vi "AO Python Interface.vi"(7 "Calling VI Ref":refnum<vi>) -> ()   [LabVIEW 2016]
uses:
  AO Python Controls/LabView Python Notifier Element.ctl
  AO Python Controls/AO Python Actions.ctl
  AO Python Controls/AO Python Data Type.ctl
  AO Python Controls/AO Python Units.ctl
  AO Python Controls/AO Python Vector Type.ctl
  Hardware Configuration/Hardware Configuration Controls/Device Type.ctl
  Hardware Configuration/Hardware Configuration Controls/Device Function.ctl
  Device Library/AOTF and AOM/AOTF Controls/AOTF Actions.ctl
panel:
  in  "Quit":bool
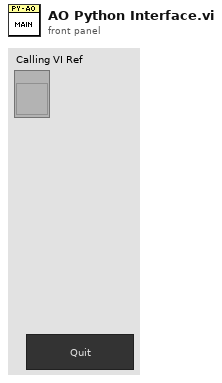
[diagram p1: front panel]
types:
  T1 = typedef "AO Python Actions.ctl" = enum16{"Error Check", "Query Commands", "Run Update", "Run Sensorless", "Wait for Command", "Get Image", "Update DM", "Get Status", "Quit"}
  T2 = typedef "LabView Python Notifier Element.ctl" = cluster{"Actions":T1, "Received?":bool, "Running?":bool, "AO Data":T3, "Command List":string[], "Python Status":string, "Error":errorcluster}
  T3 = typedef "AO Python Data Type.ctl" = cluster{"LV Command":string, "Vector":dbl[], "Flat On?":i32, "Units":T4, "Vector Type":T5}
  T4 = typedef "AO Python Units.ctl" = enum16{"rad", "nm"}
  T5 = typedef "AO Python Vector Type.ctl" = enum16{"Zernike", "Actuators", "Zernike High NA", "DM Modes"}
  T6 = typedef "Device Function.ctl" = enum16{"Primary", "Secondary", "Overview", "Wide Field Drift Correction", "642 nm Excitation", "560 nm Excitation", "546 nm Excitation", "488 nm Excitation", "405 nm Excitation", "Objective Drift Correction", "Objective XY", "Objective Z", "Sample XY", "Sample Coarse Z", "Sample Z", "4Pi Lower", "4Pi Upper", "Adj Cavity"}
  T7 = typedef "Device Type.ctl" = enum16{"AOTF", "Camera", "Deformable Mirror", "Laser", "Shutter", "Stage"}
  T8 = typedef "AOTF Actions.ctl" = enum16{"Error Check", "Blank", "Line On/Off", "Set Power", "Status", "Quit"}
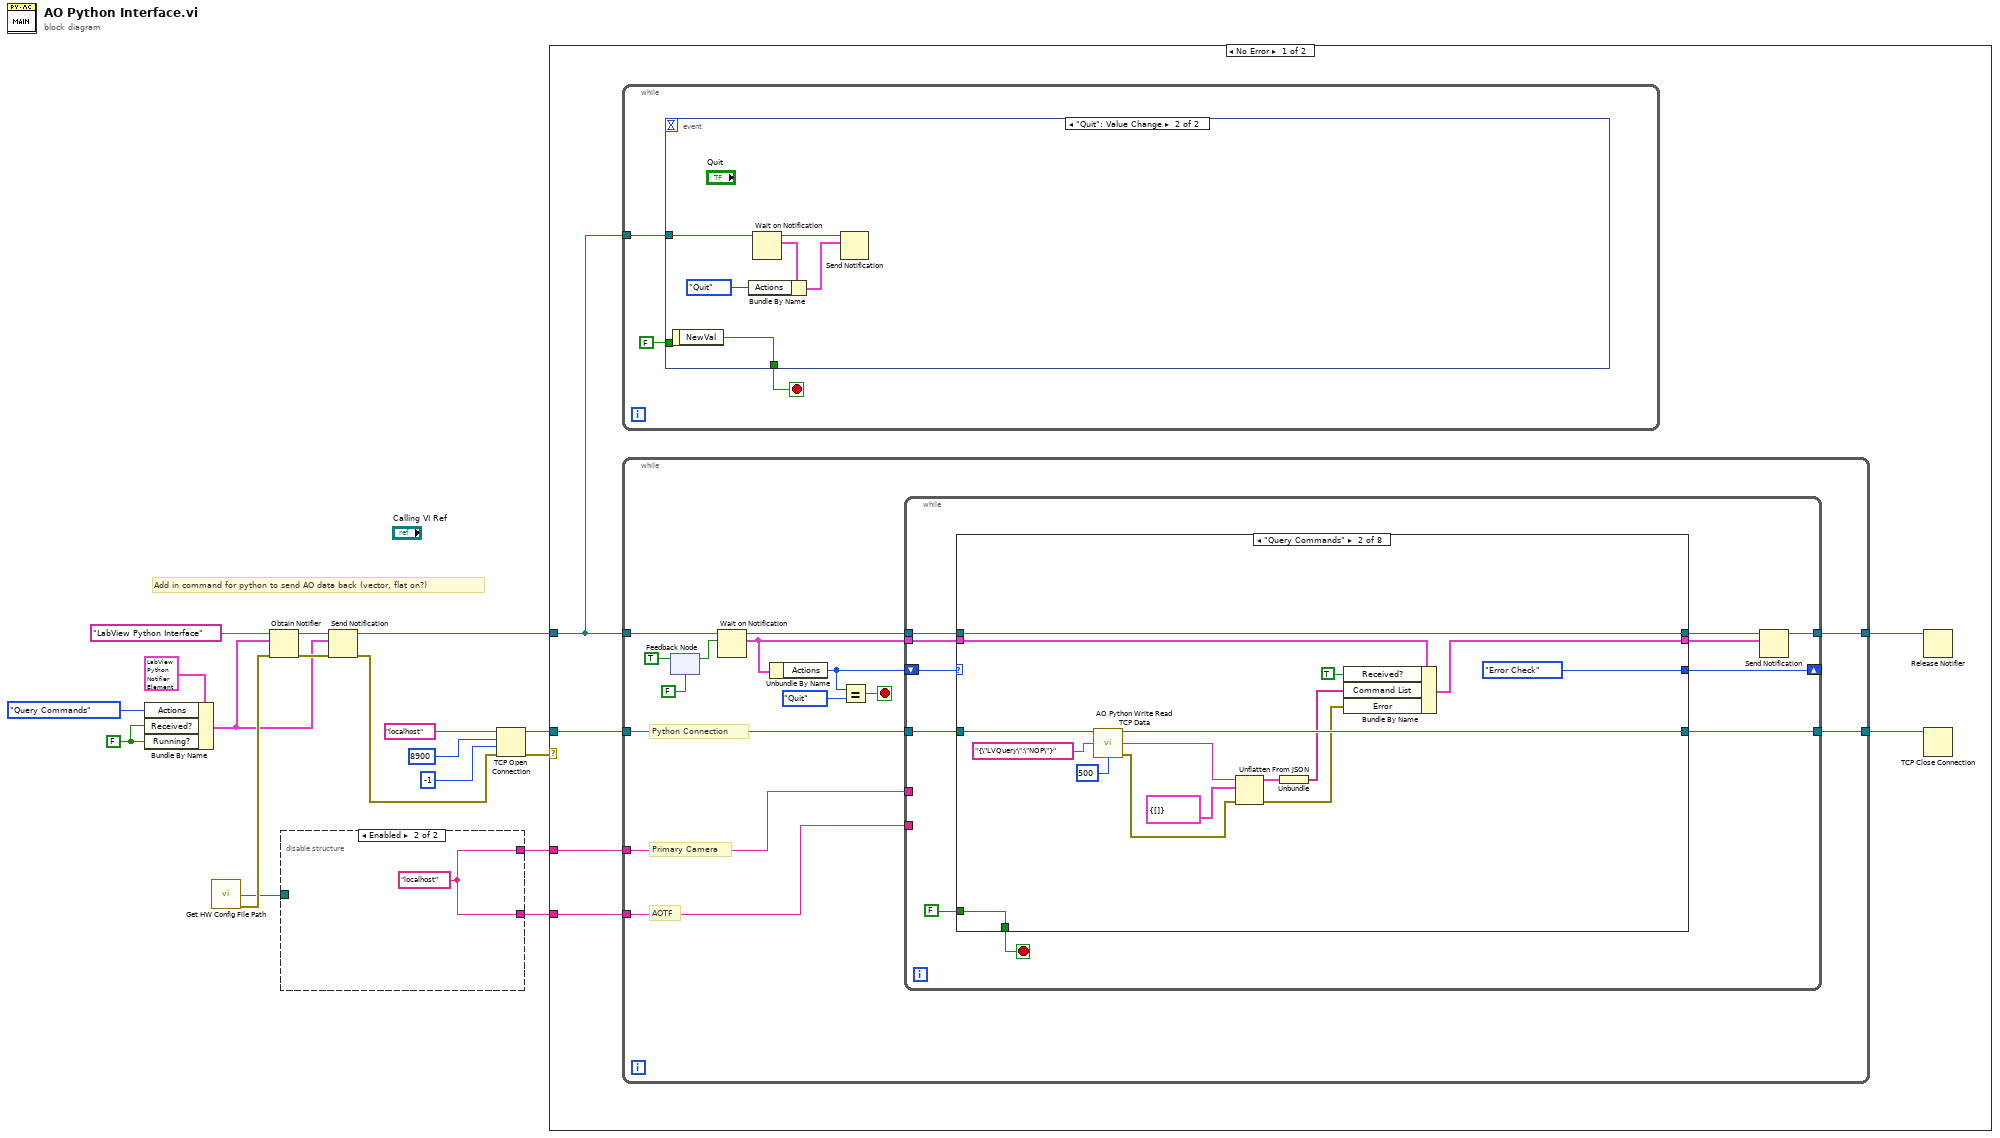
[diagram p0: block diagram]
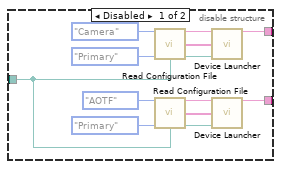
[diagram p2: hidden frame]
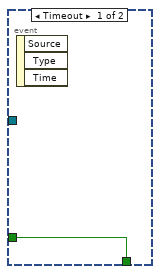
[diagram p3: hidden frame]
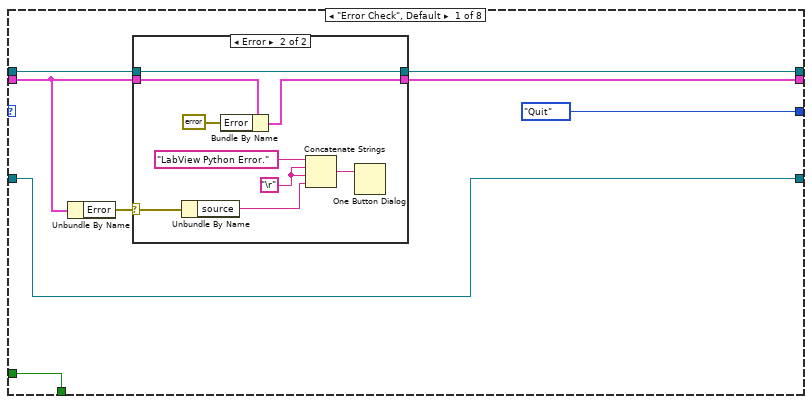
[diagram p4: hidden frame]
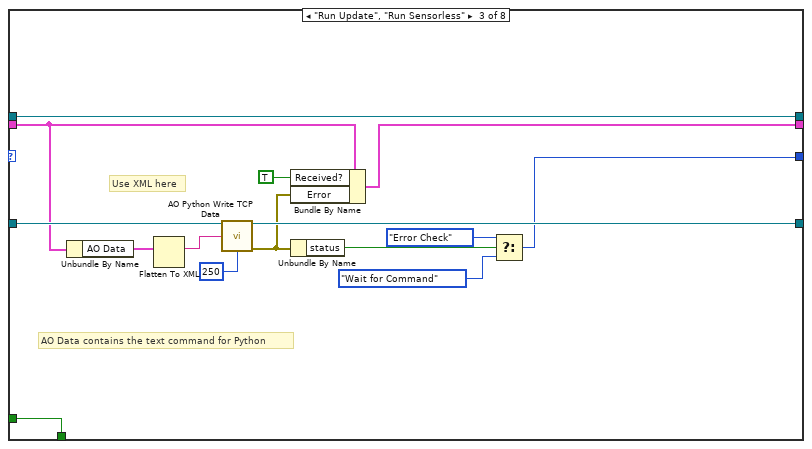
[diagram p6: hidden frame]
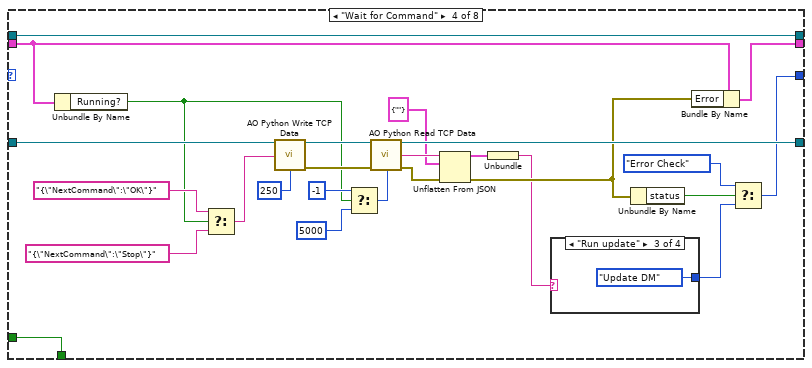
[diagram p7: hidden frame]
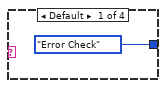
[diagram p8: hidden frame]
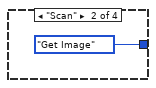
[diagram p9: hidden frame]
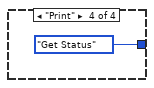
[diagram p10: hidden frame]
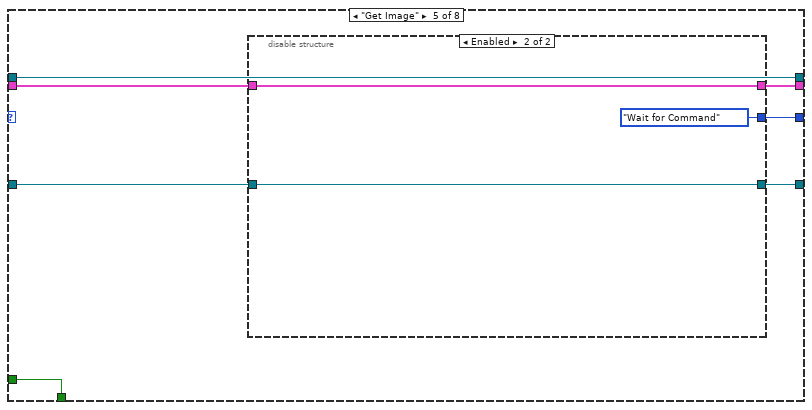
[diagram p11: hidden frame]
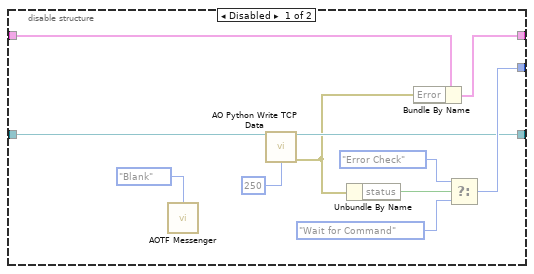
[diagram p12: hidden frame]
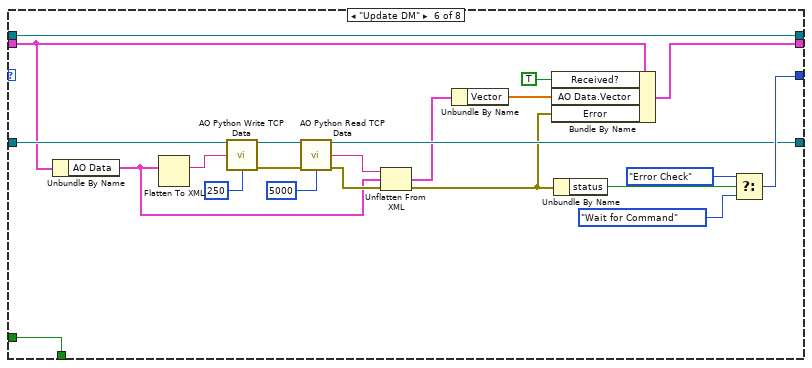
[diagram p13: hidden frame]
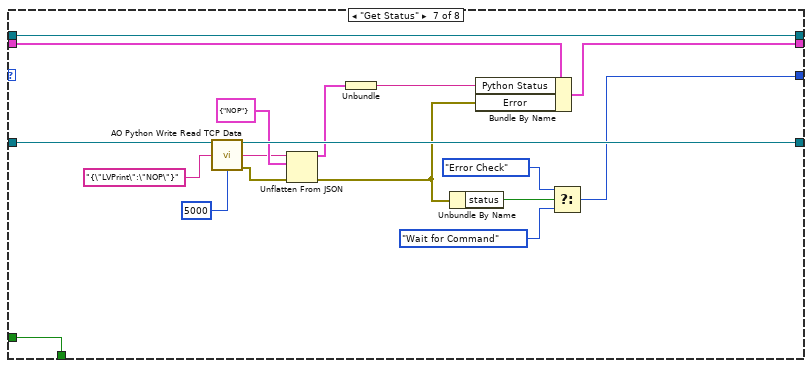
[diagram p14: hidden frame]
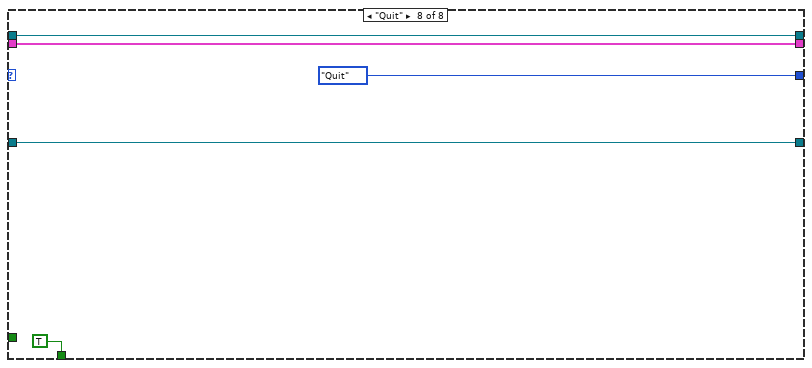
[diagram p15: hidden frame]
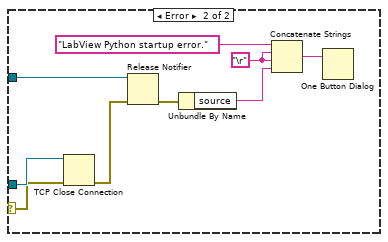
[diagram p16: hidden frame]
diagram:
  w3 = FALSE ("Received?")
  # "Add in command for python to send AO data back (vector, flat on?)"
  n1 = Bundle By Name(cluster=T2 {"Actions"=enum."Query Commands", "Received?"=FALSE, "Running?"=FALSE, "AO Data"={"LV Command"="", "Vector"=[], "Flat On?"=1, "Units"=enum."rad", "Vector Type"=enum."Zernike"}, "Command List"=[], "Python Status"="", "Error"={"status"=FALSE, "code"=0, "source"=""}} ("LabView Python Notifier Element"), "Actions"=AO_Python_Actions."Query Commands", "Received?"=w3, "Running?"=w3) -> (w1:T2)
  n2 = call "Get HW Config File Path.vi"() -> ("File Path"=w6:path, "Error"=w7:errorcluster)  [unwired: 14 in]
  n3 = Obtain Notifier(name (unnamed)="LabView Python Interface", notification data type=w1, error in (no error)=w7) -> (notifier out=w13:refnum<notifier>, error out=w11:errorcluster)  [unwired: 1 in, 1 out]
  n4 = disable-structure shown="Enabled" {
    disable-tunnel: [w26 w32] -> w8
    disable-tunnel: w6 -> [w20 _]
    disable-tunnel: [w19 w32] -> w5
    frame Disabled {
      n5 = call "Read Configuration File.vi"("Device Type"=Device_Type."Camera", "Device Function"=Device_Function."Primary", "Config File Path"=w20) -> ("Unique Notifier Name"=w31:string, "Device Ports/IDs/Channels"=w30:string[], "Device Engine Path"=w29:path)  [unwired: 9 in, 1 out]
      n6 = call "Read Configuration File.vi"("Device Type"=Device_Type."AOTF", "Device Function"=Device_Function."Primary", "Config File Path"=w20) -> ("Unique Notifier Name"=w21:string, "Device Ports/IDs/Channels"=w22:string[], "Device Engine Path"=w23:path)  [unwired: 9 in, 1 out]
      n7 = call "Device Launcher.vi"("Notifier Name"=w31, "Device Ports/IDs/Channels"=w30, "Device Engine Path"=w29) -> ("Notifier Name"=w26:string)  [unwired: 11 in, 1 out]
      n8 = call "Device Launcher.vi"("Notifier Name"=w21, "Device Ports/IDs/Channels"=w22, "Device Engine Path"=w23) -> ("Notifier Name"=w19:string)  [unwired: 11 in, 1 out]
    }
    frame Enabled {
      w32 = "localhost" ("address")
    }
  }
  n9 = Send Notification(notification=w1, notifier=w13, error in (no error)=w11) -> (notifier out=w12:refnum<notifier>, error out=w10:errorcluster)
  n10 = TCP Open Connection(address="localhost", remote port or service name=u16 8900, timeout ms (60000)=-1, error in (no error)=w10) -> (connection ID=w15:refnum<k5>, error out=w9:errorcluster)  [unwired: 1 in]
  n11 = case shown="No Error" w9 {
    selector: w9 -> [_ w226]
    tunnel: w15 -> [w38 w227]
    tunnel: w12 -> [w33 w228]
    tunnel: w8 -> [w37 _]
    tunnel: w5 -> [w34 _]
    frame No Error {
      n12 = while {
        tunnel: w33 -> [w39]
        stop <- w41 stop-if-true
        n13 = event shown="[1] \"Quit\": Value Change" {
          selector: _ -> [_ _]
          dyn-events: _ -> [_ _]
          timeout: _ -> [_ _]
          tunnel: [w42 w48] -> w41
          tunnel: FALSE -> [w42 _]
          tunnel: w39 -> [_ w47]
          event Timeout {
            n14 = event-data() -> ()  [unwired: 1 in, 3 out]
          }
          event "Quit": Value Change {
            n15 = event-data() -> ("NewVal"=w48:bool)  [unwired: 1 in]
            n16 = Wait on Notification(notifier=w47) -> (notifier out=w46:refnum<notifier>, notification=w45:T2)  [unwired: 3 in, 2 out]
            n17 = Bundle By Name(cluster=w45, "Actions"=AO_Python_Actions."Quit") -> (w43:T2)
            n18 = Send Notification(notification=w43, notifier=w46) -> ()  [unwired: 1 in, 2 out]
          }
        }
      }
      n19 = while {
        tunnel: w38 -> [w53]
        tunnel: w33 -> [w62]
        tunnel: w37 -> [w52]
        tunnel: [w51] -> w35
        tunnel: [w50] -> w36
        tunnel: w34 -> [w49]
        stop <- w58 stop-if-true
        # "AOTF"
        # "Primary Camera"
        # "Python Connection"
        n20 = feedback-in #1(TRUE) -> ()
        n21 = feedback #1(FALSE) -> (w55:bool)
        n22 = Wait on Notification(notifier=w62, ignore previous (F)=w55) -> (notifier out=w60:refnum<notifier>, notification=w54:T2)  [unwired: 2 in, 2 out]
        n23 = Unbundle By Name(w54) -> ("Actions"=w59:T1)
        n24 = Equal?(x=w59, y=AO_Python_Actions."Quit") -> (x = y?=w58:bool)
        n25 = while {
          tunnel: w60 -> [w71]
          shift-right: [w70] -> _
          shift-left: w59 -> [w73]
          tunnel: w54 -> [w72]
          tunnel: w53 -> [w68]
          tunnel: w52 -> [_]
          tunnel: [w66] -> w51
          tunnel: [w64] -> w50
          tunnel: w49 -> [_]
          stop <- w69 stop-if-true
          n26 = case shown="\"Query Commands\"" w73 {
            tunnel: w72 -> [w80 w98 w116 w133 w158 w182 w207 w215]
            tunnel: w71 -> [w81 w100 w120 w141 w159 w189 w213 w216]
            tunnel: [AO_Python_Actions."Quit" ("y") AO_Python_Actions."Error Check" ("y") w109 w134 w156 w188 w205 AO_Python_Actions."Quit" ("y")] -> w70
            tunnel: [w78 w108 w123 w149 w160 w175 w214 TRUE] -> w69
            tunnel: w68 -> [w76 w107 w122 w148 w155 w191 w212 w217]
            tunnel: FALSE -> [w78 w108 w123 w149 w160 w175 w214 _]
            tunnel: [w76 w106 w117 w136 w154 w185 w210 w217] -> w66
            tunnel: [w77 w100 w120 w141 w159 w189 w213 w216] -> w65
            tunnel: [w75 w97 w110 w132 w157 w190 w206 w215] -> w63
            frame "Error Check", Default {
              n27 = Unbundle By Name(w80) -> ("Error"=w79:errorcluster)
              n28 = case shown="Error" w79 {
                selector: w79 -> [_ w87]
                tunnel: w80 -> [w82 w91]
                tunnel: [w83 w89] -> w77
                tunnel: w81 -> [w83 w89]
                tunnel: [w82 w88] -> w75
                frame No Error {
                }
                frame Error {
                  w85 = "\r"
                  n29 = Unbundle By Name(w87) -> ("source"=w84:string)
                  n30 = Bundle By Name(cluster=w91, "Error"=errorcluster {"status"=FALSE, "code"=0, "source"=""}) -> (w88:T2)
                  n31 = Concatenate Strings("LabView Python Error." ("string"), w85, w85, w84) -> (w92:string)
                  n32 = One Button Dialog(message=w92) -> ()  [unwired: 1 in, 1 out]
                }
              }
            }
            frame "Query Commands" {
              n33 = call "AO Python Write Read TCP Data.vi"("Connection ID"=w107, "Write String"="{\"LVQuery\":\"NOP\"}", "Timeout (ms)"=500) -> ("Connection ID (Dup)"=w106:refnum<k5>, "Read String"=w101:string, "Error Out"=w99:errorcluster)  [unwired: 10 in]
              n34 = Unflatten From JSON(JSON string=w101, type and defaults=cluster{string[]} {[]}, error in (no error)=w99) -> (value=w103:cluster{string[]}, error out=w95:errorcluster)  [unwired: 4 in]
              n35 = Unbundle(w103) -> (w96:string[])
              n36 = Bundle By Name(cluster=w98, "Received?"=TRUE, "Command List"=w96, "Error"=w95) -> (w97:T2)
            }
            frame "Run Update", "Run Sensorless" {
              # "Use XML here"
              # "AO Data contains the text command for Python"
              n37 = Unbundle By Name(w116) -> ("AO Data"=w119:T3)
              n38 = Flatten To XML(anything=w119) -> (xml string=w118:string)
              n39 = call "AO Python Write TCP Data.vi"("Connection ID"=w122, "Write String"=w118, "Timeout (ms)"=250) -> ("Connection ID (Dup)"=w117:refnum<k5>, "Error Out"=w114:errorcluster)  [unwired: 11 in]
              n40 = Bundle By Name(cluster=w116, "Received?"=TRUE, "Error"=w114) -> (w110:T2)
              n41 = Unbundle By Name(w114) -> ("status"=w113:bool)
              n42 = Select(t=AO_Python_Actions."Error Check", s=w113, f=AO_Python_Actions."Wait for Command" ("y")) -> (s? t:f=w109:T1)
            }
            frame "Wait for Command" {
              n43 = Unbundle By Name(w133) -> ("Running?"=w131:bool)
              n44 = Select(t="{\"NextCommand\":\"OK\"}", s=w131, f="{\"NextCommand\":\"Stop\"}") -> (s? t:f=w142:string)
              n45 = call "AO Python Write TCP Data.vi"("Connection ID"=w148, "Write String"=w142, "Timeout (ms)"=250) -> ("Connection ID (Dup)"=w147:refnum<k5>, "Error Out"=w146:errorcluster)  [unwired: 11 in]
              n46 = Select(t=-1 ("Timeout (ms)"), s=w131, f=5000 ("Timeout (ms)")) -> (s? t:f=w137:i32)
              n47 = call "AO Python Read TCP Data.vi"("Connection ID"=w147, "Error"=w146, "Timeout (ms)"=w137) -> ("Connection ID (Dup)"=w136:refnum<k5>, "Read String"=w130:string, "Error Out"=w129:errorcluster)  [unwired: 10 in]
              n48 = Unflatten From JSON(JSON string=w130, type and defaults=cluster{string} {""}, error in (no error)=w129) -> (value=w126:cluster{string}, error out=w128:errorcluster)  [unwired: 4 in]
              n49 = Unbundle(w126) -> (w125:string)
              n50 = case shown="\"Run update\"" w125 {
                tunnel: [AO_Python_Actions."Error Check" ("y") AO_Python_Actions."Get Image" ("y") AO_Python_Actions."Update DM" ("y") AO_Python_Actions."Get Status" ("y")] -> w124
                frame Default {
                }
                frame "Scan" {
                }
                frame "Run update" {
                }
                frame "Print" {
                }
              }
              n51 = Unbundle By Name(w128) -> ("status"=w140:bool)
              n52 = Bundle By Name(cluster=w133, "Error"=w128) -> (w132:T2)
              n53 = Select(t=AO_Python_Actions."Error Check" ("y"), s=w140, f=w124) -> (s? t:f=w134:T1)
            }
            frame "Get Image" {
              n54 = disable-structure shown="Enabled" {
                disable-tunnel: w158 -> [w168 w174]
                disable-tunnel: [w167 w174] -> w157
                disable-tunnel: [w166 AO_Python_Actions."Wait for Command" ("y")] -> w156
                disable-tunnel: w155 -> [w165 w173]
                disable-tunnel: [w163 w173] -> w154
                frame Disabled {
                  n55 = call "AOTF Messenger.vi"("AOTF Action"=AOTF_Actions."Blank") -> ()  [unwired: 10 in, 5 out]
                  n56 = call "AO Python Write TCP Data.vi"("Connection ID"=w165, "Timeout (ms)"=250) -> ("Connection ID (Dup)"=w163:refnum<k5>, "Error Out"=w162:errorcluster)  [unwired: 12 in]
                  n57 = Unbundle By Name(w162) -> ("status"=w171:bool)
                  n58 = Bundle By Name(cluster=w168, "Error"=w162) -> (w167:T2)
                  n59 = Select(t=AO_Python_Actions."Error Check" ("y"), s=w171, f=AO_Python_Actions."Wait for Command" ("y")) -> (s? t:f=w166:T1)
                }
                frame Enabled {
                }
              }
            }
            frame "Update DM" {
              n60 = Unbundle By Name(w182) -> ("AO Data"=w178:T3)
              n61 = Flatten To XML(anything=w178) -> (xml string=w195:string)
              n62 = call "AO Python Write TCP Data.vi"("Connection ID"=w191, "Write String"=w195, "Timeout (ms)"=250) -> ("Connection ID (Dup)"=w186:refnum<k5>, "Error Out"=w184:errorcluster)  [unwired: 11 in]
              n63 = call "AO Python Read TCP Data.vi"("Connection ID"=w186, "Error"=w184, "Timeout (ms)"=5000) -> ("Connection ID (Dup)"=w185:refnum<k5>, "Read String"=w181:string, "Error Out"=w180:errorcluster)  [unwired: 10 in]
              n64 = Unflatten From XML(xml string=w181, type=w178, error in (no error)=w180) -> (value=w177:T3, error out=w179:errorcluster)
              n65 = Unbundle By Name(w177) -> ("Vector"=w176:dbl[])
              n66 = Bundle By Name(cluster=w182, "Received?"=TRUE, "AO Data.Vector"=w176, "Error"=w179) -> (w190:T2)
              n67 = Unbundle By Name(w179) -> ("status"=w194:bool)
              n68 = Select(t=AO_Python_Actions."Error Check", s=w194, f=AO_Python_Actions."Wait for Command" ("y")) -> (s? t:f=w188:T1)
            }
            frame "Get Status" {
              n69 = call "AO Python Write Read TCP Data.vi"("Connection ID"=w212, "Write String"="{\"LVPrint\":\"NOP\"}", "Timeout (ms)"=5000) -> ("Connection ID (Dup)"=w210:refnum<k5>, "Read String"=w201:string, "Error Out"=w200:errorcluster)  [unwired: 10 in]
              n70 = Unflatten From JSON(JSON string=w201, type and defaults=cluster{string} {"NOP"}, error in (no error)=w200) -> (value=w198:cluster{string}, error out=w199:errorcluster)  [unwired: 4 in]
              n71 = Unbundle(w198) -> (w197:string)
              n72 = Unbundle By Name(w199) -> ("status"=w209:bool)
              n73 = Bundle By Name(cluster=w207, "Python Status"=w197, "Error"=w199) -> (w206:T2)
              n74 = Select(t=AO_Python_Actions."Error Check" ("y"), s=w209, f=AO_Python_Actions."Wait for Command" ("y")) -> (s? t:f=w205:T1)
            }
            frame "Quit" {
            }
          }
          n75 = Send Notification(notification=w63, notifier=w65) -> (notifier out=w64:refnum<notifier>)  [unwired: 1 in, 1 out]
        }
      }
      n76 = Release Notifier(notifier=w36) -> ()  [unwired: 2 in, 3 out]
      n77 = TCP Close Connection(connection ID=w35) -> ()  [unwired: 2 in, 2 out]
    }
    frame Error {
      w223 = "\r"
      n78 = TCP Close Connection(connection ID=w227, error in (no error)=w226) -> (error out=w225:errorcluster)  [unwired: 1 in, 1 out]
      n79 = Release Notifier(notifier=w228, error in (no error)=w225) -> (error out=w222:errorcluster)  [unwired: 1 in, 2 out]
      n80 = Unbundle By Name(w222) -> ("source"=w221:string)
      n81 = Concatenate Strings("LabView Python startup error.", w223, w223, w221) -> (w220:string)
      n82 = One Button Dialog(message=w220) -> ()  [unwired: 1 in, 1 out]
    }
  }
